vi "Write Double.vi"(8 "error in (no error)":errorcluster, 9 "Timeout (ms)":i32, 10 "Data":dbl, 11 "CIFTag in":refnum<class "CIF_NIChn_Double.lvclass">) -> (0 "error out":errorcluster, 1 "timed out?":bool, 3 "CIFTag out":refnum<class "CIF_NIChn_Double.lvclass">)   [LabVIEW 2021, in "CIF_NIChn_Double.lvclass"]
uses:
  CIF_NIChn_Double.lvclass
  D:/dev/Packages/Channel_Manager/src/CIF_NIChn/NIChn/CIF_NIChn.lvclass
  NIChn/CIF_NIChn.lvclass/CIF_NIChn.ctl
  CIF_NIChn_Double.lvclass/CIF_NIChn_Double.ctl
  e6e5dc56-0fe0-434b-816e-55c2e61471c2.vi
  e6e5dc56-0fe0-434b-816e-55c2e61471c2.vi/4bc1c15b-36ab-481f-b8dd-c64075ce723a.vi
  e6e5dc56-0fe0-434b-816e-55c2e61471c2.vi/d83cb72b-7713-41fc-a3d1-682de79cf574.vi
  <vilib>/CIFChannels/SubVIs/Get dll Path.vi
  NIChn/CIF_NIChn.lvclass
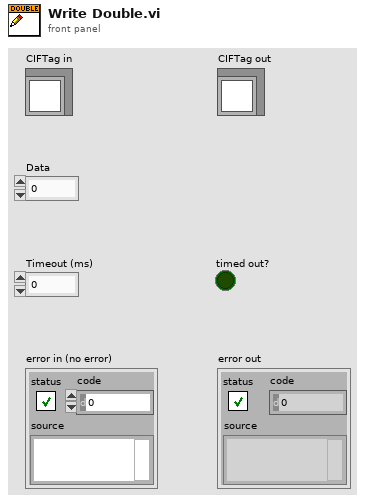
[diagram p1: front panel]
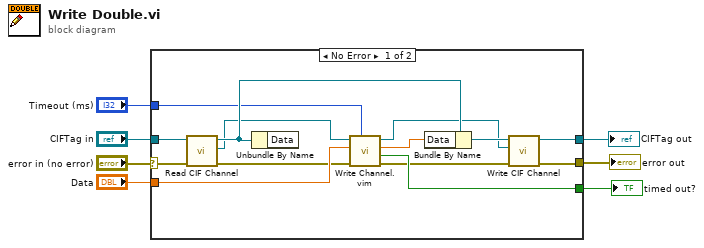
[diagram p0: block diagram]
diagram:
  n1 = case shown="No Error" "error in (no error)" {
    selector: "error in (no error)" -> [w18 w23]
    tunnel: [w12 w23] -> w6
    tunnel: [w14 w22] -> w4
    tunnel: "CIFTag in" -> [w19 w22]
    tunnel: "Data" -> [w21 _]
    tunnel: [w20 _] -> w2
    tunnel: "Timeout (ms)" -> [w9 _]
    frame No Error {
      n2 = call "Read CIF Channel.vi"("error in (no error)"=w18, "CIFTag in"=w19) -> ("error out"=w16:errorcluster, "CIF Channel"=w11:refnum<k21>, "CIFTag out"=w17:refnum<class "CIF_NIChn_Double.lvclass">)  [unwired: 7 in]
      n3 = Unbundle By Name(w17) -> ()  [unwired: 1 out]
      n4 = call "Write Channel.vim"("Timeout (ms)"=w9, "error in"=w16, "Data in"=w21, "CIF Channel in"=w11) -> ("error out"=w13:errorcluster, "Timed out?"=w20:bool, "Data out"=w8:dbl, "CIF Channel out"=w10:refnum<k21>)  [unwired: 4 in]
      n5 = Bundle By Name(cluster=w17, "Data"=w8) -> (w15:refnum<class "CIF_NIChn_Double.lvclass">)
      n6 = call "Write CIF Channel.vi"("error in (no error)"=w13, "CIF Channel"=w10, "CIFTag in"=w15) -> ("error out"=w12:errorcluster, "CIFTag out"=w14:refnum<class "CIF_NIChn_Double.lvclass">)  [unwired: 7 in]
    }
    frame Error {
    }
  }
  "error out" <- w6
  "CIFTag out" <- w4
  "timed out?" <- w2
